vi "Get VersionList From Flattened Object.vi"(9 "Number of Levels":u32, 10 "Index After ClassName":i32, 11 "Flattened Object Data":u8[](array[numeric])) -> (1 "Index After VersionList":u32, 2 "Version List":string[](array[string]))   [LabVIEW 2017, in "Composition.lvlib"]
doc: "Gets the version list for all classes from flattened object data. The first version number represents the version of the most specific child."
uses:
  Composition.lvlib
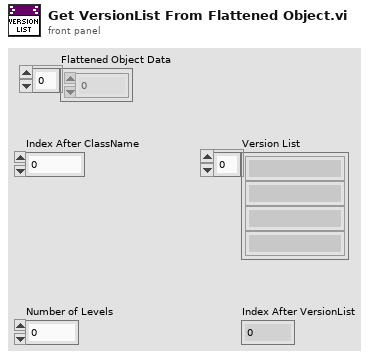
[diagram p1: front panel]
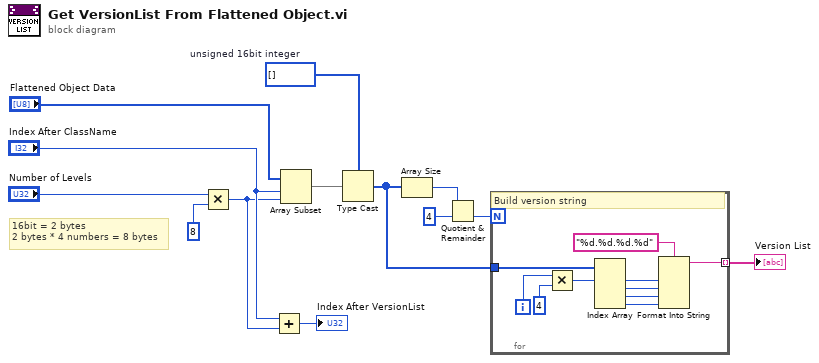
[diagram p0: block diagram]
diagram:
  w10 = u16[] []  # unsigned 16bit integer
  # "16bit = 2 bytes\n2 bytes * 4 numbers = 8 bytes"
  n1 = Multiply(x="Number of Levels", y=u32 8) -> (x*y=w3:u32)
  n2 = Add(x="Index After ClassName", y=w3) -> (x+y=→"Index After VersionList":u32)
  n3 = Array Subset(array="Flattened Object Data", index="Index After ClassName", length=w3) -> (w11:u8[])
  n4 = Type Cast(type=w10, x=w11) -> (*(type *) &x=w9:u16[])
  n5 = Array Size(array=w9) -> (size(s)=w13:i32)
  n6 = Quotient & Remainder(x=w13, y=4) -> (floor(x/y)=w7:i32)  [unwired: 1 out]
  n7 = for {
    N: w7 -> [_]
    tunnel: w9 -> [w14]
    tunnel: [w15] -> w6 mode=indexing
    i -> [w23]
    # "Build version string"
    n8 = Multiply(x=w23, y=4) -> (x*y=w21:i32)
    n9 = Index Array(array=w14, index #1=w21) -> (element #1=w19:u16, element #2=w18:u16, element #3=w17:u16, element #4=w16:u16)  [unwired: 3 in]
    n10 = Format Into String(format string="%d.%d.%d.%d", w19, w18, w17, w16) -> (resulting string=w15:string)  [unwired: 2 in, 1 out]
  }
  "Version List" <- w6
